vi "Pos ctrl window-Initialise.vi"(8 "error in (no error)":errorcluster, 9 "Pos ctrl window refs":T1) -> (0 "error out":errorcluster, 3 "XYZ movement ctrl window queue ref":refnum<queue>)   [LabVIEW 2020]
uses:
  Typedefs/Pos Ctrl queue data cluster.ctl
  Typedefs/Pos Ctrl States.ctl
  Typedefs/Pos Ctrl window refs cluster.ctl
  <userlib>/My Palettes.lib/Custom Controls/Directional Arrow Buttons/Arrow button-North.ctl
  Globals/Pos ctrl window globals.vi
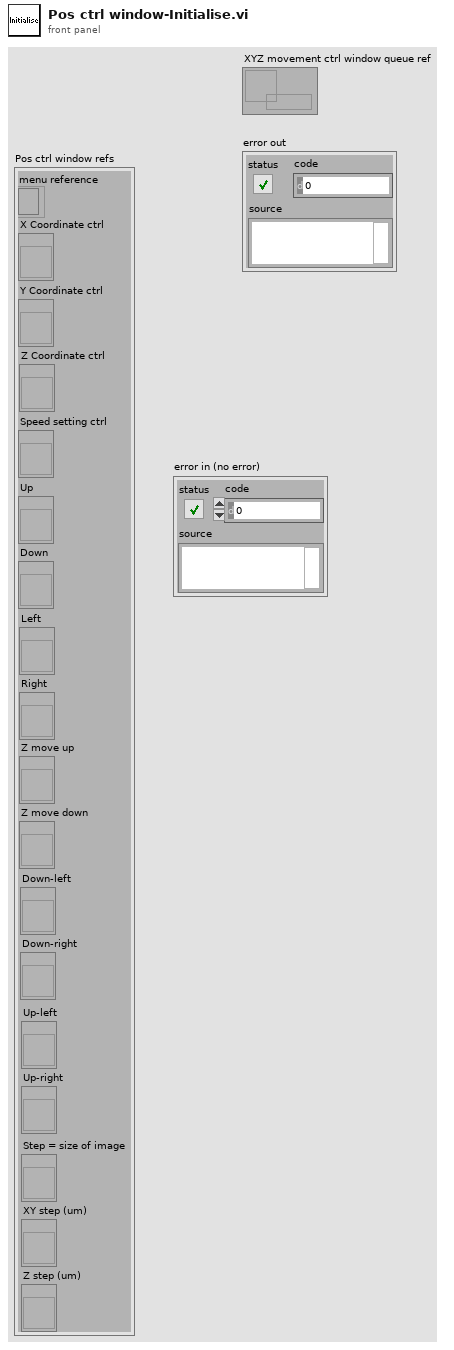
[diagram p1: front panel]
types:
  T1 = typedef "Pos Ctrl window refs cluster.ctl" = cluster{"menu reference":refnum<k9>, "X Coordinate ctrl":refnum<vi>, "Y Coordinate ctrl":refnum<vi>, "Z Coordinate ctrl":refnum<vi>, "Speed setting ctrl":refnum<vi>, "Up":refnum<vi>, "Down":refnum<vi>, "Left":refnum<vi>, "Right":refnum<vi>, "Z move up":refnum<vi>, "Z move down":refnum<vi>, "Down-left":refnum<vi>, "Down-right":refnum<vi>, "Up-left":refnum<vi>, "Up-right":refnum<vi>, "Step = size of image":refnum<vi>, "XY step (um)":refnum<vi>, "Z step (um)":refnum<vi>}
  T2 = enum8{"Enabled", "Disabled", "Disabled and Grayed Out"}
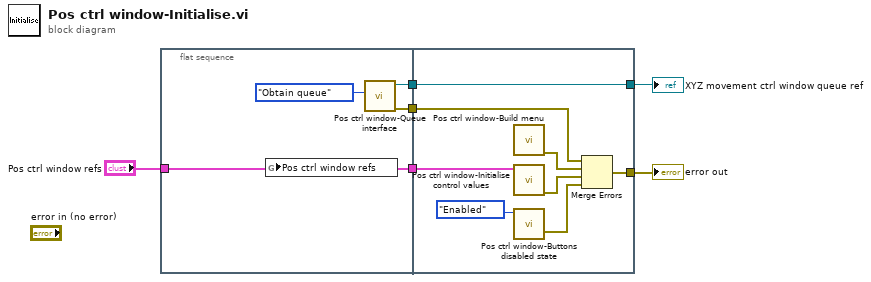
[diagram p0: block diagram]
diagram:
  n1 = flat-sequence {
    tunnel: "Pos ctrl window refs" -> [w7]
    tunnel: [w7] -> w3
    tunnel: [w9] -> w2
    tunnel: [w8] -> w1
    tunnel: [w12] -> w5
    tunnel: [w15] -> w4
    tunnel: w3 -> [w18]
    tunnel: w2 -> [w12]
    tunnel: w1 -> [w11]
    frame #0 {
      n2 = global write "Pos ctrl window globals.vi" "Pos ctrl window refs"(w7) -> ()
      n3 = call "Pos ctrl window-Queue interface.vi"("Function"=enum16{"None", "Release queue", "Obtain queue"}."Obtain queue") -> ("error out"=w8:errorcluster, "Pos ctrl window queue"=w9:refnum<queue>)  [unwired: 9 in]
    }
    frame #1 {
      n4 = call "Pos ctrl window-Build menu.vi"() -> ("error out"=w14:errorcluster)  [unwired: 10 in, 1 out]
      n5 = call "Pos ctrl window-Initialise control values.vi"("Pos ctrl window refs"=w18) -> ("error out"=w13:errorcluster)  [unwired: 10 in]
      n6 = call "Pos ctrl window-Buttons disabled state.vi"("Disabled"=T2."Enabled") -> ("error out"=w16:errorcluster)  [unwired: 10 in]
      n7 = Merge Errors(w11, w14, w13, w16) -> (w15:errorcluster)
    }
  }
  "error out" <- w4
  "XYZ movement ctrl window queue ref" <- w5
